vi "Get Image Data.vi"(8 "error in (no error)":errorcluster, 11 "path to PNG file":path) -> (0 "error out":errorcluster, 2 "image data":T1)   [LabVIEW 2020]
uses:
  <vilib>/picture/picture.llb/imagedata.ctl
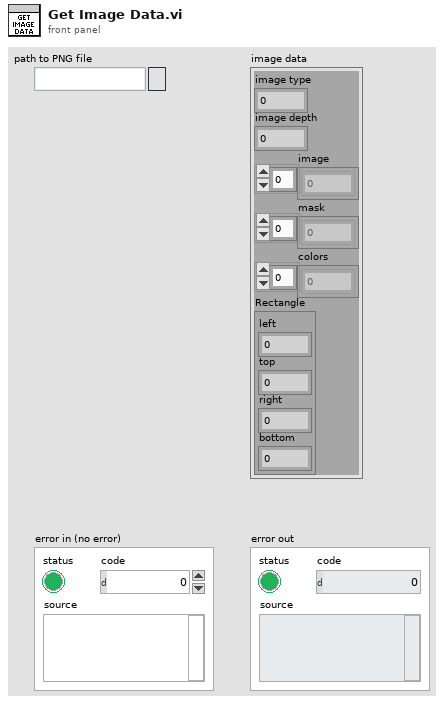
[diagram p1: front panel]
types:
  T1 = typedef "imagedata.ctl" = cluster{"image type":i32, "image depth":i32, "image":u8[], "mask":u8[], "colors":u32[], "Rectangle":cluster{"left":i16, "top":i16, "right":i16, "bottom":i16}}
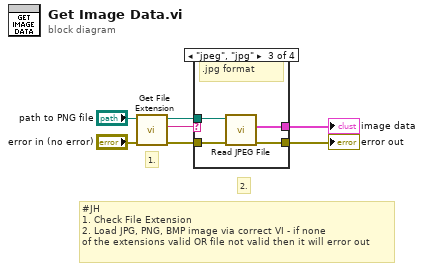
[diagram p0: block diagram]
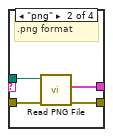
[diagram p3: hidden frame]
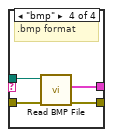
[diagram p4: hidden frame]
diagram:
  # "#JH\n1. Check File Extension\n2. Load JPG, PNG, BMP image via correct VI - if none\nof the extensions valid OR file not valid then it will error out"
  # "2."
  # "1."
  n1 = call <vilib>:"Get File Extension.vi"("error in (no error)"="error in (no error)", "file"="path to PNG file") -> ("error out"=w6:errorcluster, "lowercase file extension"=w4:string, "dup file"=w7:path)  [unwired: 5 in, 2 out]
  n2 = case shown="\"jpeg\", \"jpg\"" w4 {
    tunnel: [w8 w12 w15 w19] -> w1
    tunnel: w6 -> [w8 w11 w16 w20]
    tunnel: [_ w10 w13 w17] -> w2
    tunnel: w7 -> [_ w9 w14 w18]
    frame Default {
    }
    frame "png" {
      # ".png format"
      n3 = call <vilib>:"Read PNG File.vi"("error in (no error)"=w11, "path to PNG file"=w9) -> ("error out"=w12:errorcluster, "image data"=w10:T1)  [unwired: 7 in, 1 out]
    }
    frame "jpeg", "jpg" {
      # ".jpg format"
      n4 = call <vilib>:"Read JPEG File.vi"("error in (no error)"=w16, "path to JPEG file"=w14) -> ("error out"=w15:errorcluster, "image data"=w13:T1)  [unwired: 7 in, 1 out]
    }
    frame "bmp" {
      # ".bmp format"
      n5 = call <vilib>:"Read BMP File.vi"("error in (no error)"=w20, "path to BMP file"=w18) -> ("error out"=w19:errorcluster, "image data"=w17:T1)  [unwired: 7 in, 1 out]
    }
  }
  "image data" <- w2
  "error out" <- w1
